vi "Assertion Failure Message.vi"() -> ()   [LabVIEW 2017, in "Assertion.Tests.lvlib" / "Assert Error Code.lvlib"]
uses:
  Assert Error Code.lvlib
  <vilib>/Utility/error.llb/Error Cluster From Error Code.vi
  <vilib>/ErrorRing/Error Ring.xnode
  Assertion/Assertion.lvlib
panel:
  out "error out":errorcluster
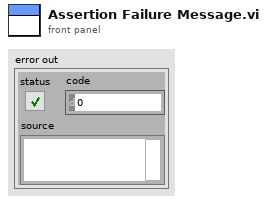
[diagram p1: front panel]
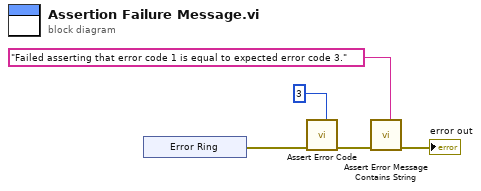
[diagram p0: block diagram]
diagram:
  n1 = xnode "Error Ring"() -> ("error out"=w5:errorcluster)
  n2 = call "Assert Error Code.vi"("Expected"=3, "error in (no error)"=w5) -> ("error out"=w1:errorcluster)  [unwired: 9 in]
  n3 = call "Assert Error Message Contains String.vi"("Expected"="Failed asserting that error code 1 is equal to expected error code 3." ("Needle"), "error in (no error)"=w1) -> ("error out"=→"error out":errorcluster)  [unwired: 9 in]
